vi "sub vi - Read Analog All v9.5.vi"(0 "data 0":waveform(dbl)[](array[waveform]), 5 "data 1":waveform(dbl)[](array[waveform]), 7 "data 2":waveform(dbl)[](array[waveform]), 9 "AI Error":errorcluster[](array[cluster])) -> (3 "array GRAPH":dynamicdata[](array[waveform]), 4 "LAB01":T2, 6 "LAB02":T3, 8 "LAB03":T4, 10 "LAB04":T5, 13 "deg C":dbl, 14 "USB Error":bool[](array[boolean]), 15 "LAB05":T6)   [LabVIEW 2017]
uses:
  program files/Global display 3.vi
  <vilib>/measure/mascope.llb/Amplitude and Levels 1 chan.vi
  <vilib>/measure/NI_MAPro.lvlib
  <vilib>/measure/madcrms.llb/Basic Averaged DC-RMS for N Chan.vi
panel:
  in  "normalized waveform":waveform(dbl)
  in  "Tab Control":T1(tab)
  out "LAB01-2 (PF)":dbl
  out "LAB01-1 (PF)":dbl
  out "LAB01-2 (V)":dbl
  out "LAB01-2 (A)":dbl
  out "LAB01-1 (V)":dbl
  out "LAB01-1 (A)":dbl
  out "LAB01-2 (GRAPH)":dynamicdata(graph)
  out "LAB01-1 (GRAPH)":dynamicdata(graph)
  out "LAB02-2 (PF)":dbl
  out "LAB02-1 (PF)":dbl
  out "LAB02-2 (V)":dbl
  out "LAB02-2 (A)":dbl
  out "LAB02-1 (V)":dbl
  out "LAB02-1 (A)":dbl
  out "LAB02-2 (GRAPH)":dynamicdata(graph)
  out "LAB02-1 (GRAPH)":dynamicdata(graph)
  out "LAB03-2 (PF)":dbl
  out "LAB03-1 (PF)":dbl
  out "LAB03-2 (V)":dbl
  out "LAB03-2 (A)":dbl
  out "LAB03-1 (V)":dbl
  out "LAB03-1 (A)":dbl
  out "LAB03-2 (GRAPH)":dynamicdata(graph)
  out "LAB03-1 (GRAPH)":dynamicdata(graph)
  out "LAB04-2 (PF)":dbl
  out "LAB04-1 (PF)":dbl
  out "LAB04-2 (V)":dbl
  out "LAB04-2 (A)":dbl
  out "LAB04-1 (V)":dbl
  out "LAB04-1 (A)":dbl
  out "LAB04-1 (GRAPH)":dynamicdata(graph)
  out "LAB04-2 (GRAPH)":dynamicdata(graph)
  out "LAB05-2 (PF)":dbl
  out "LAB05-1 (PF)":dbl
  out "LAB05-2 (V)":dbl
  out "LAB05-2 (A)":dbl
  out "LAB05-1 (V)":dbl
  out "LAB05-1 (A)":dbl
  out "LAB05-1 (GRAPH)":dynamicdata(graph)
  out "LAB05-2 (GRAPH)":dynamicdata(graph)
  out "A1 error":errorcluster
  out "array ERROR":errorcluster[](array[cluster])
  out "AI2-OFF":waveform(dbl)[](graph)
  out "AI2-ON":waveform(dbl)[](graph)
  out "AI1-OFF":waveform(dbl)[](graph)
  out "AI1-ON":waveform(dbl)[](graph)
  out "AI0-OFF":waveform(dbl)[](graph)
  out "AI0-ON":waveform(dbl)[](graph)
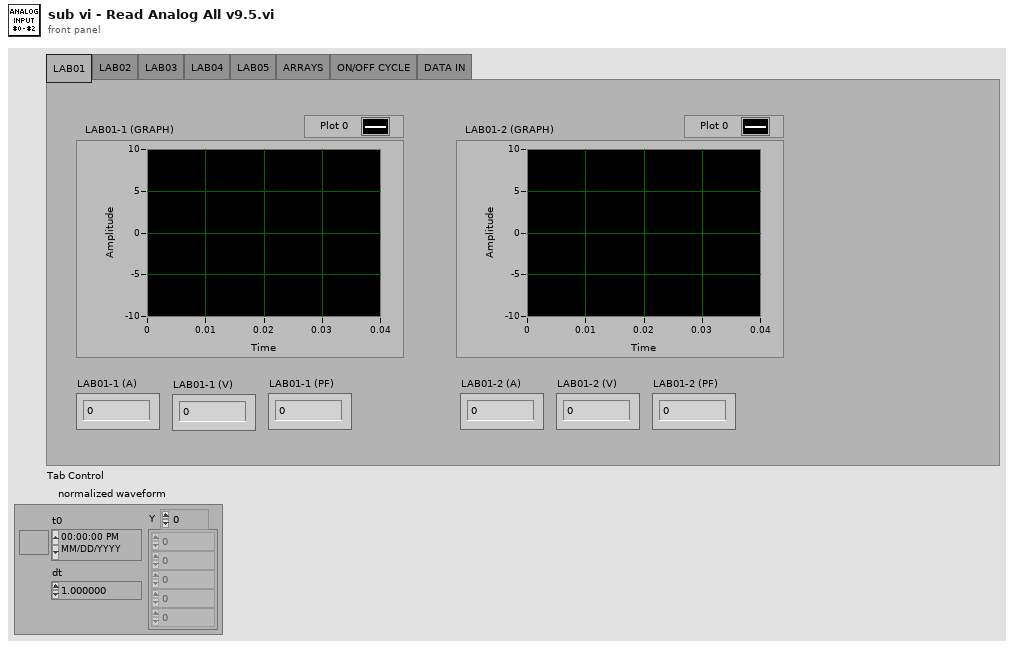
[diagram p1: front panel]
types:
  T1 = enum32{"LAB01", "LAB02", "LAB03", "LAB04", "LAB05", "ARRAYS", "ON/OFF CYCLE", "DATA IN"}
  T2 = cluster{"LAB01-1 (A)":dbl, "LAB01-1 (V)":dbl, "LAB01-1 (PF)":dbl, "LAB01-2 (A)":dbl, "LAB01-2 (V)":dbl, "LAB01-2 (PF)":dbl}
  T3 = cluster{"LAB02-1 (A)":dbl, "LAB02-1 (V)":dbl, "LAB02-1 (PF)":dbl, "LAB02-2 (A)":dbl, "LAB02-2 (V)":dbl, "LAB02-2 (PF)":dbl}
  T4 = cluster{"LAB03-1 (A)":dbl, "LAB03-1 (V)":dbl, "LAB03-1 (PF)":dbl, "LAB03-2 (A)":dbl, "LAB03-2 (V)":dbl, "LAB03-2 (PF)":dbl}
  T5 = cluster{"LAB04-1 (A)":dbl, "LAB04-1 (V)":dbl, "LAB04-1 (PF)":dbl, "LAB04-2 (A)":dbl, "LAB04-2 (V)":dbl, "LAB04-2 (PF)":dbl}
  T6 = cluster{"LAB05-1 (A)":dbl, "LAB05-1 (V)":dbl, "LAB05-1 (PF)":dbl, "LAB05-2 (A)":dbl, "LAB05-2 (V)":dbl, "LAB05-2 (PF)":dbl}
  T7 = cluster{"active power [W]":dbl, "apparent power [VA]":dbl, "reactive power [VAR]":dbl, "power factor":dbl}
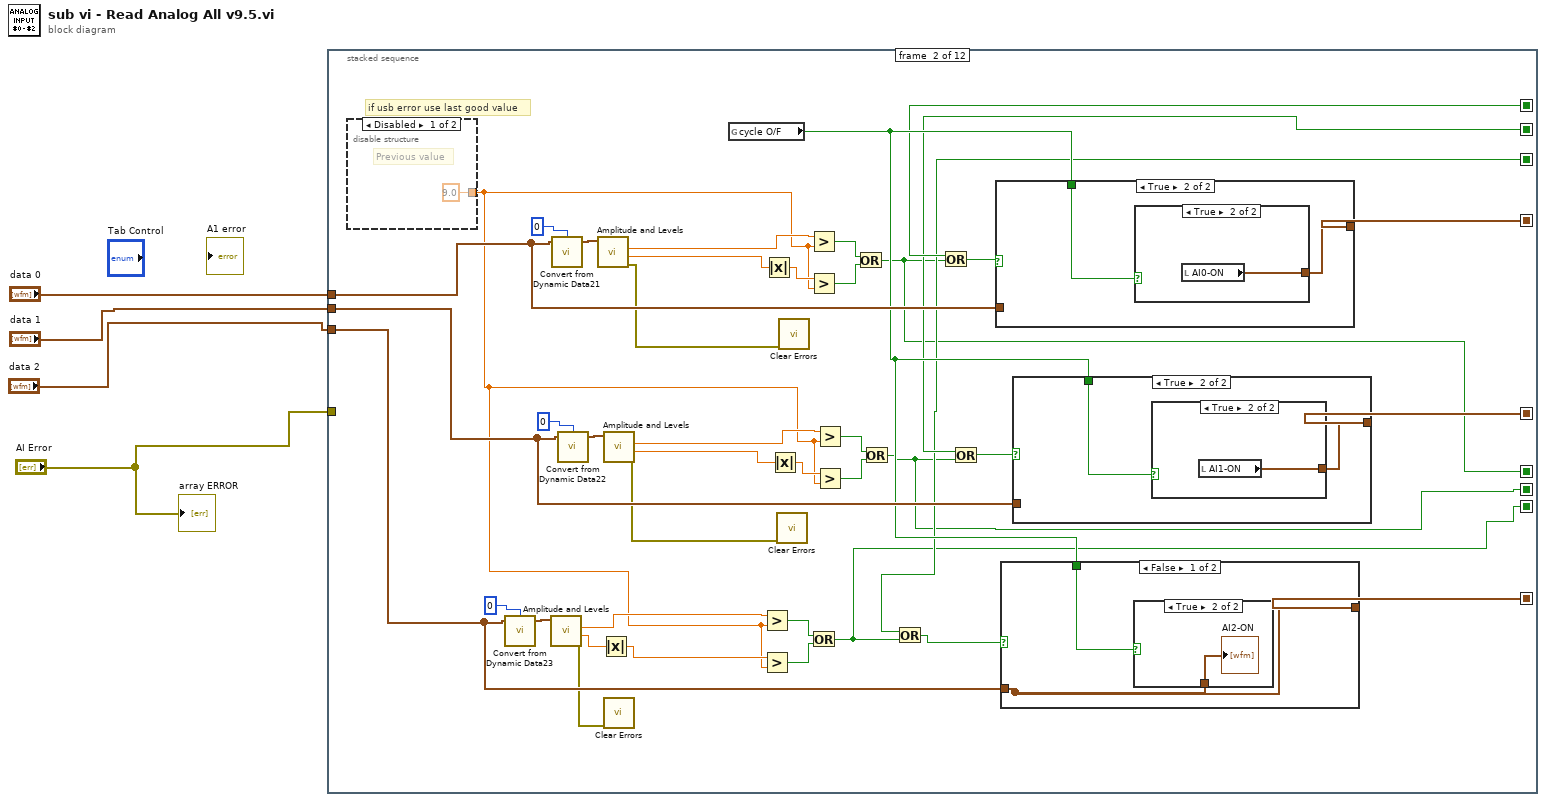
[diagram p0: block diagram]
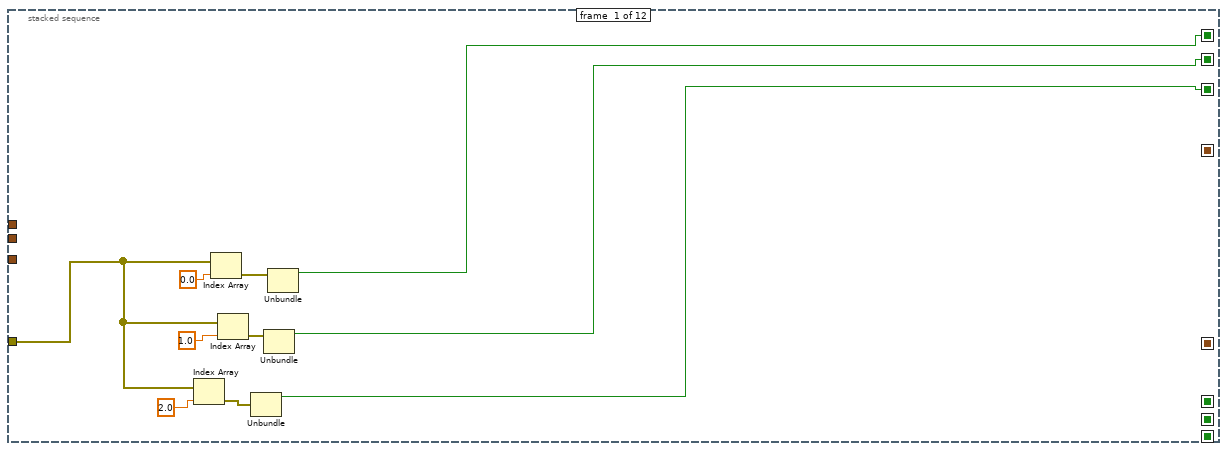
[diagram p2: hidden frame]
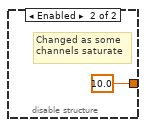
[diagram p3: hidden frame]
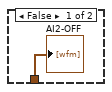
[diagram p4: hidden frame]
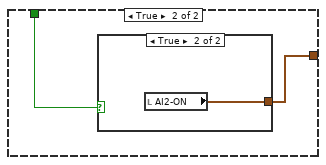
[diagram p5: hidden frame]
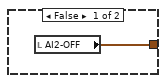
[diagram p6: hidden frame]
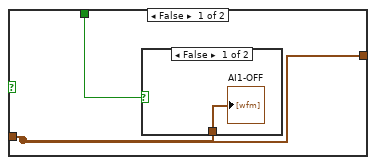
[diagram p7: hidden frame]
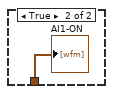
[diagram p8: hidden frame]
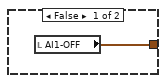
[diagram p9: hidden frame]
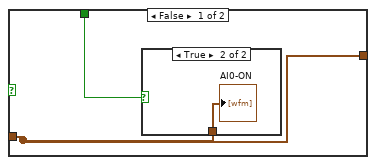
[diagram p10: hidden frame]
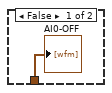
[diagram p11: hidden frame]
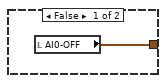
[diagram p12: hidden frame]
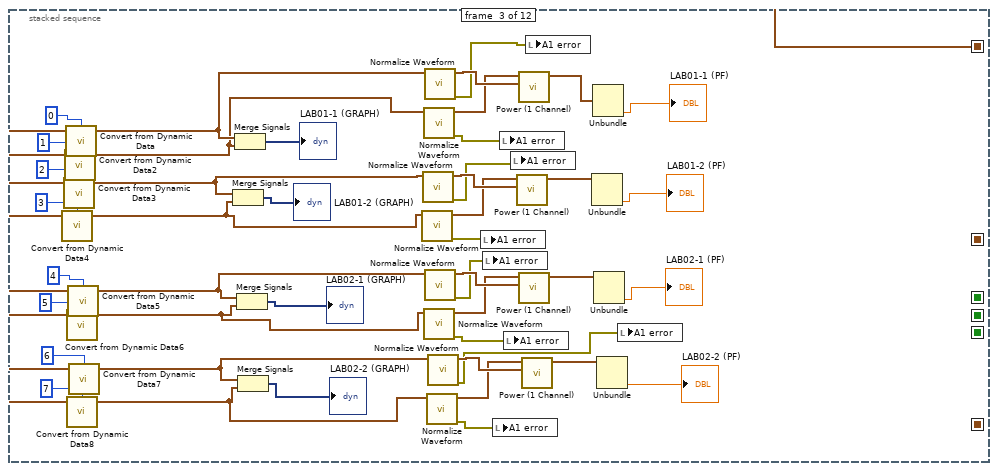
[diagram p13: hidden frame]
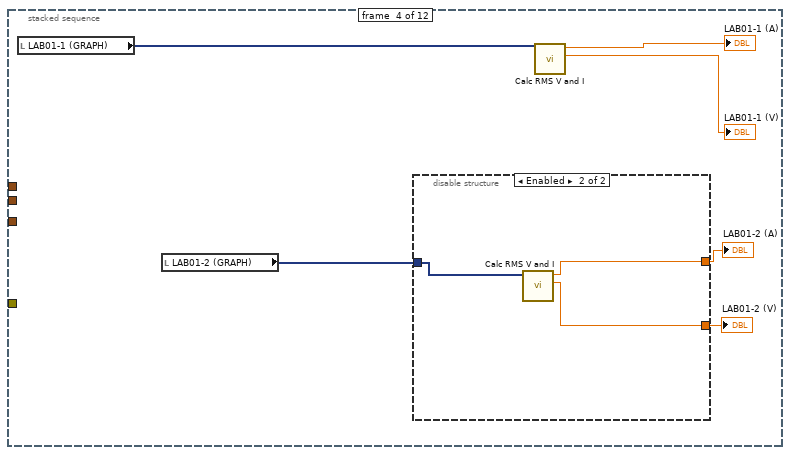
[diagram p14: hidden frame]
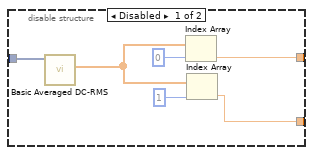
[diagram p15: hidden frame]
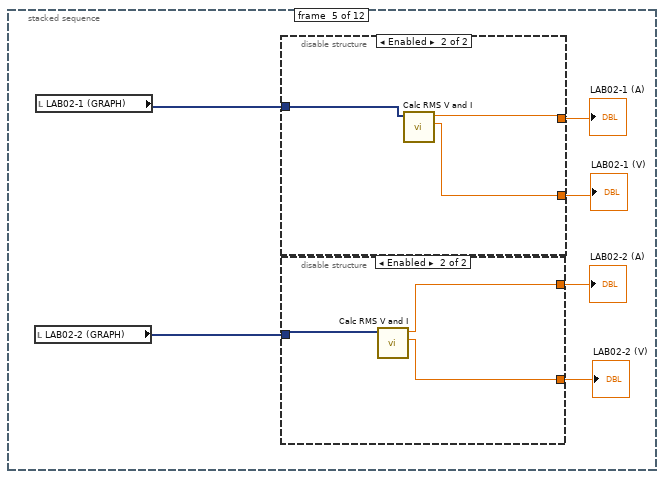
[diagram p16: hidden frame]
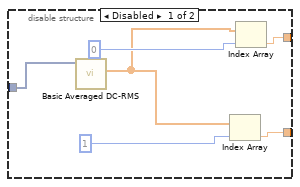
[diagram p17: hidden frame]
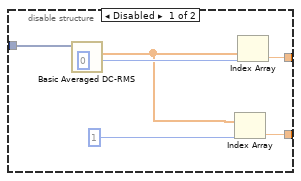
[diagram p18: hidden frame]
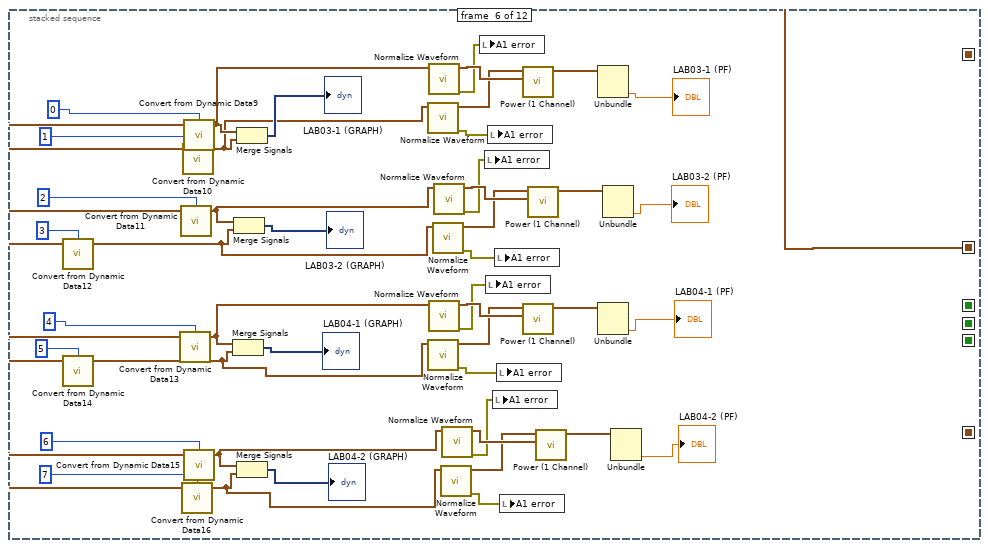
[diagram p19: hidden frame]
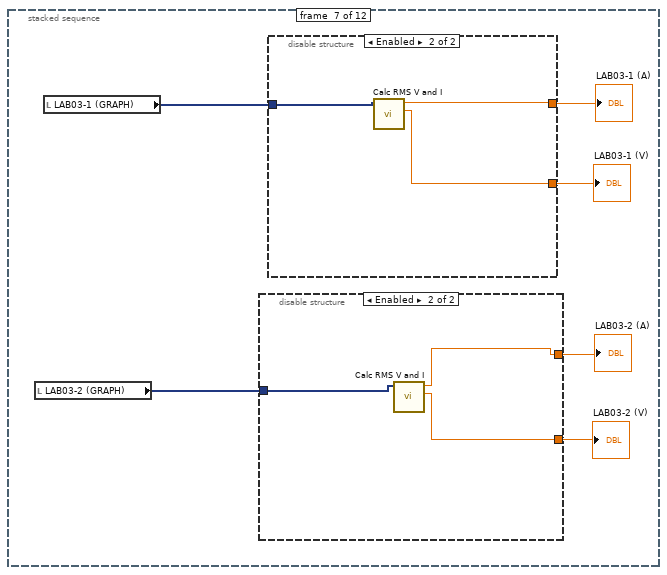
[diagram p20: hidden frame]
diagram:
  n1 = stacked-sequence {
    seq-local: [w12 _ _ _ _ _ _ _ _ _ _ _] -> [_ w22 _ _ _ _ _ _ _ _ _ w325]
    seq-local: [w9 _ _ _ _ _ _ _ _ _ _ _] -> [_ w21 _ _ _ _ _ _ _ _ _ w324]
    seq-local: [w5 _ _ _ _ _ _ _ _ _ _ _] -> [_ w18 _ _ _ _ _ _ _ _ _ w323]
    seq-local: [_ w48 _ _ _ _ _ _ _ _ _ _] -> [_ _ w126 _ _ _ _ _ _ _ _ _]
    seq-local: [_ w38 _ _ _ _ _ _ _ _ _ _] -> [_ _ _ _ _ w210 _ _ _ _ _ _]
    seq-local: [_ w27 _ _ _ _ _ _ _ _ _ _] -> [_ _ _ _ _ _ _ _ w261 _ _ _]
    seq-local: [_ w17 _ _ _ _ _ _ _ _ _ _] -> [_ _ _ _ _ _ _ _ _ _ _ w322]
    seq-local: [_ w16 _ _ _ _ _ _ _ _ _ _] -> [_ _ _ _ _ _ _ _ _ _ _ w321]
    seq-local: [_ w15 _ _ _ _ _ _ _ _ _ _] -> [_ _ _ _ _ _ _ _ _ _ _ w320]
    tunnel: "data 0" -> [_ w47 _ _ _ _ _ _ _ _ _ _]
    tunnel: "data 1" -> [_ w39 _ _ _ _ _ _ _ _ _ _]
    tunnel: "data 2" -> [_ w30 _ _ _ _ _ _ _ _ _ _]
    tunnel: "AI Error" -> [w6 _ _ _ _ _ _ _ _ _ _ _]
    frame #0 {
      n2 = Index Array(array=w6, index=2.0) -> (element=w7:errorcluster)
      n3 = Index Array(array=w6, index=0.0) -> (element=w13:errorcluster)
      n4 = Index Array(array=w6, index=1.0) -> (element=w10:errorcluster)
      n5 = Unbundle(w7) -> ("status"=w5:bool)  [unwired: 2 out]
      n6 = Unbundle(w10) -> ("status"=w9:bool)  [unwired: 2 out]
      n7 = Unbundle(w13) -> ("status"=w12:bool)  [unwired: 2 out]
    }
    frame #1 {
      # "if usb error use last good value"
      n8 = disable-structure shown="Disabled" {
        disable-tunnel: [9.0 10.0] -> w29
        frame Disabled {
          # "Previous value"
        }
        frame Enabled {
          # "Changed as some\nchannels saturate"
        }
      }
      n9 = call "Convert from Dynamic Data23"("Dynamic Data Type"=w30, "Channel"=0) -> ("Waveform"=w36:waveform(dbl))  [unwired: 2 in]
      n10 = call-poly <vilib>:"Amplitude and Levels.vi"("signal in"=w36) -> ("error out"=w24:errorcluster, "low state level"=w35:dbl, "high state level"=w34:dbl)  [unwired: 7 in, 1 out]
      n11 = call "Convert from Dynamic Data21"("Dynamic Data Type"=w47, "Channel"=0) -> ("Waveform"=w54:waveform(dbl))  [unwired: 2 in]
      n12 = call "Convert from Dynamic Data22"("Dynamic Data Type"=w39, "Channel"=0) -> ("Waveform"=w45:waveform(dbl))  [unwired: 2 in]
      n13 = call-poly <vilib>:"Amplitude and Levels.vi"("signal in"=w54) -> ("error out"=w26:errorcluster, "low state level"=w53:dbl, "high state level"=w52:dbl)  [unwired: 7 in, 1 out]
      n14 = Absolute Value(x=w35) -> (abs(x)=w33:dbl)
      n15 = call-poly <vilib>:"Amplitude and Levels.vi"("signal in"=w45) -> ("error out"=w25:errorcluster, "low state level"=w44:dbl, "high state level"=w43:dbl)  [unwired: 7 in, 1 out]
      n16 = call <vilib>:"Clear Errors.vi"("error in (no error)"=w24) -> ()  [unwired: 5 in, 2 out]
      n17 = global read "Global display 3.vi" "cycle O/F"() -> (w28:bool)
      n18 = Greater?(x=w34, y=w29) -> (0:w32:bool)
      n19 = Greater?(x=w33, y=w29) -> (0:w31:bool)
      n20 = Absolute Value(x=w53) -> (abs(x)=w51:dbl)
      n21 = Absolute Value(x=w44) -> (abs(x)=w42:dbl)
      n22 = call <vilib>:"Clear Errors.vi"("error in (no error)"=w25) -> ()  [unwired: 5 in, 2 out]
      n23 = call <vilib>:"Clear Errors.vi"("error in (no error)"=w26) -> ()  [unwired: 5 in, 2 out]
      n24 = Greater?(x=w52, y=w29) -> (0:w50:bool)
      n25 = Greater?(x=w51, y=w29) -> (0:w49:bool)
      n26 = Or(x=w32, y=w31) -> (x .or. y?=w15:bool)
      n27 = Greater?(x=w43, y=w29) -> (0:w41:bool)
      n28 = Greater?(x=w42, y=w29) -> (0:w40:bool)
      n29 = Or(x=w50, y=w49) -> (x .or. y?=w17:bool)
      n30 = Or(x=w41, y=w40) -> (x .or. y?=w16:bool)
      n31 = Or(x=w18, y=w15) -> (x .or. y?=w19:bool)
      n32 = Or(x=w22, y=w17) -> (x .or. y?=w23:bool)
      n33 = Or(x=w21, y=w16) -> (x .or. y?=w20:bool)
      n34 = case shown="True" w23 {
        tunnel: w28 -> [w75 w79]
        tunnel: [w74 w78] -> w48
        tunnel: w47 -> [w74 _]
        frame False {
          n35 = case shown="True" w75 {
            tunnel: w74 -> [w76 w77]
            frame False {
              "AI0-OFF" <- w76
            }
            frame True {
              "AI0-ON" <- w77
            }
          }
        }
        frame True {
          n36 = case shown="True" w79 {
            tunnel: [w80 w81] -> w78
            frame False {
              n37 = local read "AI0-OFF"() -> (w80:waveform(dbl)[])
            }
            frame True {
              n38 = local read "AI0-ON"() -> (w81:waveform(dbl)[])
            }
          }
        }
      }
      n39 = case shown="False" w19 {
        tunnel: w28 -> [w59 w63]
        tunnel: [w58 w62] -> w27
        tunnel: w30 -> [w58 _]
        frame False {
          n40 = case shown="True" w59 {
            tunnel: w58 -> [w60 w61]
            frame False {
              "AI2-OFF" <- w60
            }
            frame True {
              "AI2-ON" <- w61
            }
          }
        }
        frame True {
          n41 = case shown="True" w63 {
            tunnel: [w64 w65] -> w62
            frame False {
              n42 = local read "AI2-OFF"() -> (w64:waveform(dbl)[])
            }
            frame True {
              n43 = local read "AI2-ON"() -> (w65:waveform(dbl)[])
            }
          }
        }
      }
      n44 = case shown="True" w20 {
        tunnel: w28 -> [w67 w71]
        tunnel: [w66 w70] -> w38
        tunnel: w39 -> [w66 _]
        frame False {
          n45 = case shown="False" w67 {
            tunnel: w66 -> [w68 w69]
            frame False {
              "AI1-OFF" <- w68
            }
            frame True {
              "AI1-ON" <- w69
            }
          }
        }
        frame True {
          n46 = case shown="True" w71 {
            tunnel: [w72 w73] -> w70
            frame False {
              n47 = local read "AI1-OFF"() -> (w72:waveform(dbl)[])
            }
            frame True {
              n48 = local read "AI1-ON"() -> (w73:waveform(dbl)[])
            }
          }
        }
      }
    }
    frame #2 {
      n49 = call "Convert from Dynamic Data4"("Dynamic Data Type"=w126, "Channel"=3) -> ("Waveform"=w102:waveform(dbl))  [unwired: 2 in]
      n50 = call "Convert from Dynamic Data3"("Dynamic Data Type"=w126, "Channel"=2) -> ("Waveform"=w103:waveform(dbl))  [unwired: 2 in]
      n51 = call "Convert from Dynamic Data2"("Dynamic Data Type"=w126, "Channel"=1) -> ("Waveform"=w112:waveform(dbl))  [unwired: 2 in]
      n52 = call "Convert from Dynamic Data"("Dynamic Data Type"=w126, "Channel"=0) -> ("Waveform"=w113:waveform(dbl))  [unwired: 2 in]
      n53 = call "Convert from Dynamic Data6"("Dynamic Data Type"=w126, "Channel"=5) -> ("Waveform"=w97:waveform(dbl))  [unwired: 2 in]
      n54 = call "Convert from Dynamic Data8"("Dynamic Data Type"=w126, "Channel"=7) -> ("Waveform"=w91:waveform(dbl))  [unwired: 2 in]
      n55 = call "Convert from Dynamic Data5"("Dynamic Data Type"=w126, "Channel"=4) -> ("Waveform"=w98:waveform(dbl))  [unwired: 2 in]
      n56 = call "Convert from Dynamic Data7"("Dynamic Data Type"=w126, "Channel"=6) -> ("Waveform"=w92:waveform(dbl))  [unwired: 2 in]
      n57 = Merge Signals(w103, w102) -> (→"LAB01-2 (GRAPH)":dynamicdata)
      n58 = Merge Signals(w113, w112) -> (→"LAB01-1 (GRAPH)":dynamicdata)
      n59 = Merge Signals(w98, w97) -> (→"LAB02-1 (GRAPH)":dynamicdata)
      n60 = Merge Signals(w92, w91) -> (→"LAB02-2 (GRAPH)":dynamicdata)
      n61 = call <vilib>:"Normalize Waveform.vi"("waveform in"=w102) -> ("error out"=w86:errorcluster, "normalized waveform"=w106:waveform(dbl))  [unwired: 7 in, 2 out]
      n62 = call <vilib>:"Normalize Waveform.vi"("waveform in"=w103) -> ("error out"=w87:errorcluster, "normalized waveform"=w107:waveform(dbl))  [unwired: 7 in, 2 out]
      n63 = call <vilib>:"Normalize Waveform.vi"("waveform in"=w112) -> ("error out"=w88:errorcluster, "normalized waveform"=w110:waveform(dbl))  [unwired: 7 in, 2 out]
      n64 = call <vilib>:"Normalize Waveform.vi"("waveform in"=w97) -> ("error out"=w84:errorcluster, "normalized waveform"=w100:waveform(dbl))  [unwired: 7 in, 2 out]
      n65 = call <vilib>:"Normalize Waveform.vi"("waveform in"=w113) -> ("error out"=w89:errorcluster, "normalized waveform"=w111:waveform(dbl))  [unwired: 7 in, 2 out]
      n66 = call <vilib>:"Normalize Waveform.vi"("waveform in"=w98) -> ("error out"=w85:errorcluster, "normalized waveform"=w101:waveform(dbl))  [unwired: 7 in, 2 out]
      n67 = call <vilib>:"Normalize Waveform.vi"("waveform in"=w91) -> ("error out"=w82:errorcluster, "normalized waveform"=w94:waveform(dbl))  [unwired: 7 in, 2 out]
      n68 = call <vilib>:"Normalize Waveform.vi"("waveform in"=w92) -> ("error out"=w83:errorcluster, "normalized waveform"=w95:waveform(dbl))  [unwired: 7 in, 2 out]
      n69 = local write "A1 error"(w86) -> ()
      n70 = local write "A1 error"(w85) -> ()
      n71 = local write "A1 error"(w82) -> ()
      n72 = local write "A1 error"(w88) -> ()
      n73 = local write "A1 error"(w84) -> ()
      n74 = local write "A1 error"(w87) -> ()
      n75 = call "Power (1 Channel).vi"("current waveform"=w107, "voltage waveform"=w106) -> ("power value"=w105:T7)  [unwired: 9 in]
      n76 = call "Power (1 Channel).vi"("current waveform"=w111, "voltage waveform"=w110) -> ("power value"=w109:T7)  [unwired: 9 in]
      n77 = call "Power (1 Channel).vi"("current waveform"=w101, "voltage waveform"=w100) -> ("power value"=w99:T7)  [unwired: 9 in]
      n78 = call "Power (1 Channel).vi"("current waveform"=w95, "voltage waveform"=w94) -> ("power value"=w93:T7)  [unwired: 9 in]
      n79 = local write "A1 error"(w89) -> ()
      n80 = Unbundle(w105) -> ("power factor"=→"LAB01-2 (PF)":dbl)  [unwired: 3 out]
      n81 = Unbundle(w109) -> ("power factor"=→"LAB01-1 (PF)":dbl)  [unwired: 3 out]
      n82 = Unbundle(w99) -> ("power factor"=→"LAB02-1 (PF)":dbl)  [unwired: 3 out]
      n83 = Unbundle(w93) -> ("power factor"=→"LAB02-2 (PF)":dbl)  [unwired: 3 out]
      n84 = local write "A1 error"(w83) -> ()
    }
    frame #3 {
      n85 = local read "LAB01-1 (GRAPH)"() -> (w127:dynamicdata)
      n86 = local read "LAB01-2 (GRAPH)"() -> (w128:dynamicdata)
      n87 = disable-structure shown="Enabled" {
        disable-tunnel: [w135 w140] -> w132
        disable-tunnel: [w134 w139] -> w131
        disable-tunnel: w128 -> [w133 w141]
        frame Disabled {
          n88 = call-poly <vilib>:"Basic Averaged DC-RMS.vi"("signals in"=w133) -> ("RMS values"=w138:dbl[])  [unwired: 7 in, 3 out]
          n89 = Index Array(array=w138, index=0) -> (element=w135:dbl)
          n90 = Index Array(array=w138, index=1) -> (element=w134:dbl)
        }
        frame Enabled {
          n91 = call "Calc RMS V and I.vi"("LAB01-1 (GRAPH)"=w141) -> ("RMS V"=w139:dbl, "RMS I"=w140:dbl)  [unwired: 9 in]
        }
      }
      "LAB01-2 (A)" <- w132
      "LAB01-2 (V)" <- w131
      n92 = call "Calc RMS V and I.vi"("LAB01-1 (GRAPH)"=w127) -> ("RMS V"=→"LAB01-1 (V)":dbl, "RMS I"=→"LAB01-1 (A)":dbl)  [unwired: 9 in]
    }
    frame #4 {
      n93 = local read "LAB02-2 (GRAPH)"() -> (w143:dynamicdata)
      n94 = local read "LAB02-1 (GRAPH)"() -> (w142:dynamicdata)
      n95 = disable-structure shown="Enabled" {
        disable-tunnel: [w159 w164] -> w147
        disable-tunnel: [w158 w163] -> w146
        disable-tunnel: w142 -> [w157 w165]
        frame Disabled {
          n96 = call-poly <vilib>:"Basic Averaged DC-RMS.vi"("signals in"=w157) -> ("RMS values"=w160:dbl[])  [unwired: 7 in, 3 out]
          n97 = Index Array(array=w160, index=1) -> (element=w158:dbl)
          n98 = Index Array(array=w160, index=0) -> (element=w159:dbl)
        }
        frame Enabled {
          n99 = call "Calc RMS V and I.vi"("LAB01-1 (GRAPH)"=w165) -> ("RMS V"=w163:dbl, "RMS I"=w164:dbl)  [unwired: 9 in]
        }
      }
      "LAB02-1 (A)" <- w147
      "LAB02-1 (V)" <- w146
      n100 = disable-structure shown="Enabled" {
        disable-tunnel: [w150 w155] -> w145
        disable-tunnel: [w149 w154] -> w144
        disable-tunnel: w143 -> [w148 w156]
        frame Disabled {
          n101 = call-poly <vilib>:"Basic Averaged DC-RMS.vi"("signals in"=w148) -> ("RMS values"=w151:dbl[])  [unwired: 7 in, 3 out]
          n102 = Index Array(array=w151, index=1) -> (element=w149:dbl)
          n103 = Index Array(array=w151, index=0) -> (element=w150:dbl)
        }
        frame Enabled {
          n104 = call "Calc RMS V and I.vi"("LAB01-1 (GRAPH)"=w156) -> ("RMS V"=w154:dbl, "RMS I"=w155:dbl)  [unwired: 9 in]
        }
      }
      "LAB02-2 (A)" <- w145
      "LAB02-2 (V)" <- w144
    }
    frame #5 {
      n105 = call "Convert from Dynamic Data12"("Dynamic Data Type"=w210, "Channel"=3) -> ("Waveform"=w187:waveform(dbl))  [unwired: 2 in]
      n106 = call "Convert from Dynamic Data14"("Dynamic Data Type"=w210, "Channel"=5) -> ("Waveform"=w181:waveform(dbl))  [unwired: 2 in]
      n107 = call "Convert from Dynamic Data13"("Dynamic Data Type"=w210, "Channel"=4) -> ("Waveform"=w182:waveform(dbl))  [unwired: 2 in]
      n108 = call "Convert from Dynamic Data11"("Dynamic Data Type"=w210, "Channel"=2) -> ("Waveform"=w188:waveform(dbl))  [unwired: 2 in]
      n109 = call "Convert from Dynamic Data16"("Dynamic Data Type"=w210, "Channel"=7) -> ("Waveform"=w175:waveform(dbl))  [unwired: 2 in]
      n110 = call "Convert from Dynamic Data10"("Dynamic Data Type"=w210, "Channel"=1) -> ("Waveform"=w193:waveform(dbl))  [unwired: 2 in]
      n111 = call "Convert from Dynamic Data9"("Dynamic Data Type"=w210, "Channel"=0) -> ("Waveform"=w194:waveform(dbl))  [unwired: 2 in]
      n112 = call "Convert from Dynamic Data15"("Dynamic Data Type"=w210, "Channel"=6) -> ("Waveform"=w176:waveform(dbl))  [unwired: 2 in]
      n113 = Merge Signals(w182, w181) -> (→"LAB04-1 (GRAPH)":dynamicdata)
      n114 = Merge Signals(w188, w187) -> (→"LAB03-2 (GRAPH)":dynamicdata)
      n115 = Merge Signals(w194, w193) -> (→"LAB03-1 (GRAPH)":dynamicdata)
      n116 = Merge Signals(w176, w175) -> (→"LAB04-2 (GRAPH)":dynamicdata)
      n117 = call <vilib>:"Normalize Waveform.vi"("waveform in"=w193) -> ("error out"=w172:errorcluster, "normalized waveform"=w196:waveform(dbl))  [unwired: 7 in, 2 out]
      n118 = call <vilib>:"Normalize Waveform.vi"("waveform in"=w181) -> ("error out"=w168:errorcluster, "normalized waveform"=w184:waveform(dbl))  [unwired: 7 in, 2 out]
      n119 = call <vilib>:"Normalize Waveform.vi"("waveform in"=w194) -> ("error out"=w173:errorcluster, "normalized waveform"=w197:waveform(dbl))  [unwired: 7 in, 2 out]
      n120 = call <vilib>:"Normalize Waveform.vi"("waveform in"=w182) -> ("error out"=w169:errorcluster, "normalized waveform"=w185:waveform(dbl))  [unwired: 7 in, 2 out]
      n121 = call <vilib>:"Normalize Waveform.vi"("waveform in"=w187) -> ("error out"=w170:errorcluster, "normalized waveform"=w190:waveform(dbl))  [unwired: 7 in, 2 out]
      n122 = call <vilib>:"Normalize Waveform.vi"("waveform in"=w188) -> ("error out"=w171:errorcluster, "normalized waveform"=w191:waveform(dbl))  [unwired: 7 in, 2 out]
      n123 = call <vilib>:"Normalize Waveform.vi"("waveform in"=w175) -> ("error out"=w166:errorcluster, "normalized waveform"=w178:waveform(dbl))  [unwired: 7 in, 2 out]
      n124 = call <vilib>:"Normalize Waveform.vi"("waveform in"=w176) -> ("error out"=w167:errorcluster, "normalized waveform"=w179:waveform(dbl))  [unwired: 7 in, 2 out]
      n125 = local write "A1 error"(w173) -> ()
      n126 = local write "A1 error"(w171) -> ()
      n127 = local write "A1 error"(w169) -> ()
      n128 = local write "A1 error"(w172) -> ()
      n129 = local write "A1 error"(w167) -> ()
      n130 = local write "A1 error"(w170) -> ()
      n131 = local write "A1 error"(w168) -> ()
      n132 = local write "A1 error"(w166) -> ()
      n133 = call "Power (1 Channel).vi"("current waveform"=w197, "voltage waveform"=w196) -> ("power value"=w195:T7)  [unwired: 9 in]
      n134 = call "Power (1 Channel).vi"("current waveform"=w185, "voltage waveform"=w184) -> ("power value"=w183:T7)  [unwired: 9 in]
      n135 = call "Power (1 Channel).vi"("current waveform"=w191, "voltage waveform"=w190) -> ("power value"=w189:T7)  [unwired: 9 in]
      n136 = call "Power (1 Channel).vi"("current waveform"=w179, "voltage waveform"=w178) -> ("power value"=w177:T7)  [unwired: 9 in]
      n137 = Unbundle(w195) -> ("power factor"=→"LAB03-1 (PF)":dbl)  [unwired: 3 out]
      n138 = Unbundle(w183) -> ("power factor"=→"LAB04-1 (PF)":dbl)  [unwired: 3 out]
      n139 = Unbundle(w189) -> ("power factor"=→"LAB03-2 (PF)":dbl)  [unwired: 3 out]
      n140 = Unbundle(w177) -> ("power factor"=→"LAB04-2 (PF)":dbl)  [unwired: 3 out]
    }
    frame #6 {
      n141 = local read "LAB03-2 (GRAPH)"() -> (w211:dynamicdata)
      n142 = local read "LAB03-1 (GRAPH)"() -> (w212:dynamicdata)
      n143 = disable-structure shown="Enabled" {
        disable-tunnel: [w219 w223] -> w214
        disable-tunnel: [w218 w224] -> w213
        disable-tunnel: w211 -> [w217 w225]
        frame Disabled {
          n144 = call-poly <vilib>:"Basic Averaged DC-RMS.vi"("signals in"=w217) -> ("RMS values"=w220:dbl[])  [unwired: 7 in, 3 out]
          n145 = Index Array(array=w220, index=0) -> (element=w218:dbl)
          n146 = Index Array(array=w220, index=1) -> (element=w219:dbl)
        }
        frame Enabled {
          n147 = call "Calc RMS V and I.vi"("LAB01-1 (GRAPH)"=w225) -> ("RMS V"=w223:dbl, "RMS I"=w224:dbl)  [unwired: 9 in]
        }
      }
      "LAB03-2 (A)" <- w213
      "LAB03-2 (V)" <- w214
      n148 = disable-structure shown="Enabled" {
        disable-tunnel: [w228 w233] -> w216
        disable-tunnel: [w227 w232] -> w215
        disable-tunnel: w212 -> [w226 w234]
        frame Disabled {
          n149 = call-poly <vilib>:"Basic Averaged DC-RMS.vi"("signals in"=w226) -> ("RMS values"=w229:dbl[])  [unwired: 7 in, 3 out]
          n150 = Index Array(array=w229, index=0) -> (element=w228:dbl)
          n151 = Index Array(array=w229, index=1) -> (element=w227:dbl)
        }
        frame Enabled {
          n152 = call "Calc RMS V and I.vi"("LAB01-1 (GRAPH)"=w234) -> ("RMS V"=w232:dbl, "RMS I"=w233:dbl)  [unwired: 9 in]
        }
      }
      "LAB03-1 (A)" <- w216
      "LAB03-1 (V)" <- w215
    }
    frame #7 {
      n153 = local read "LAB04-2 (GRAPH)"() -> (w235:dynamicdata)
      n154 = local read "LAB04-1 (GRAPH)"() -> (w236:dynamicdata)
      n155 = disable-structure shown="Enabled" {
        disable-tunnel: [w243 w247] -> w238
        disable-tunnel: [w242 w248] -> w237
        disable-tunnel: w235 -> [w241 w249]
        frame Disabled {
          n156 = call-poly <vilib>:"Basic Averaged DC-RMS.vi"("signals in"=w241) -> ("RMS values"=w244:dbl[])  [unwired: 7 in, 3 out]
          n157 = Index Array(array=w244, index=0) -> (element=w242:dbl)
          n158 = Index Array(array=w244, index=1) -> (element=w243:dbl)
        }
        frame Enabled {
          n159 = call "Calc RMS V and I.vi"("LAB01-1 (GRAPH)"=w249) -> ("RMS V"=w247:dbl, "RMS I"=w248:dbl)  [unwired: 9 in]
        }
      }
      "LAB04-2 (A)" <- w237
      "LAB04-2 (V)" <- w238
      n160 = disable-structure shown="Enabled" {
        disable-tunnel: [w252 w257] -> w240
        disable-tunnel: [w251 w256] -> w239
        disable-tunnel: w236 -> [w250 w258]
        frame Disabled {
          n161 = call-poly <vilib>:"Basic Averaged DC-RMS.vi"("signals in"=w250) -> ("RMS values"=w253:dbl[])  [unwired: 7 in, 3 out]
          n162 = Index Array(array=w253, index=0) -> (element=w252:dbl)
          n163 = Index Array(array=w253, index=1) -> (element=w251:dbl)
        }
        frame Enabled {
          n164 = call "Calc RMS V and I.vi"("LAB01-1 (GRAPH)"=w258) -> ("RMS V"=w256:dbl, "RMS I"=w257:dbl)  [unwired: 9 in]
        }
      }
      "LAB04-1 (A)" <- w240
      "LAB04-1 (V)" <- w239
    }
    frame #8 {
      n165 = call "Convert from Dynamic Data18"("Dynamic Data Type"=w261, "Channel"=1) -> ("Waveform"=w275:waveform(dbl))  [unwired: 2 in]
      n166 = call "Convert from Dynamic Data20"("Dynamic Data Type"=w261, "Channel"=3) -> ("Waveform"=w269:waveform(dbl))  [unwired: 2 in]
      n167 = call "Convert from Dynamic Data17"("Dynamic Data Type"=w261, "Channel"=0) -> ("Waveform"=w276:waveform(dbl))  [unwired: 2 in]
      n168 = call "Convert from Dynamic Data19"("Dynamic Data Type"=w261, "Channel"=2) -> ("Waveform"=w270:waveform(dbl))  [unwired: 2 in]
      n169 = Merge Signals(w276, w275) -> (→"LAB05-1 (GRAPH)":dynamicdata)
      n170 = Merge Signals(w270, w269) -> (→"LAB05-2 (GRAPH)":dynamicdata)
      n171 = call "Convert from Dynamic Data24"("Dynamic Data Type"=w261, "Channel"=4) -> ("Waveform"=w260:waveform(dbl))  [unwired: 2 in]
      n172 = call "RMS.vi"("current waveform"=w260) -> ("RMS"=→"deg C":dbl)  [unwired: 10 in]
      n173 = call <vilib>:"Normalize Waveform.vi"("waveform in"=w275) -> ("error out"=w267:errorcluster, "normalized waveform"=w277:waveform(dbl))  [unwired: 7 in, 2 out]
      n174 = call <vilib>:"Normalize Waveform.vi"("waveform in"=w276) -> ("error out"=w266:errorcluster, "normalized waveform"=w278:waveform(dbl))  [unwired: 7 in, 2 out]
      n175 = call <vilib>:"Normalize Waveform.vi"("waveform in"=w269) -> ("error out"=w265:errorcluster, "normalized waveform"=w272:waveform(dbl))  [unwired: 7 in, 2 out]
      n176 = call <vilib>:"Normalize Waveform.vi"("waveform in"=w270) -> ("error out"=w264:errorcluster, "normalized waveform"=w273:waveform(dbl))  [unwired: 7 in, 2 out]
      n177 = local write "A1 error"(w265) -> ()
      n178 = local write "A1 error"(w266) -> ()
      n179 = local write "A1 error"(w264) -> ()
      n180 = call "Power (1 Channel).vi"("current waveform"=w278, "voltage waveform"=w277) -> ("power value"=w262:T7)  [unwired: 9 in]
      n181 = local write "A1 error"(w267) -> ()
      n182 = call "Power (1 Channel).vi"("current waveform"=w273, "voltage waveform"=w272) -> ("power value"=w271:T7)  [unwired: 9 in]
      n183 = Unbundle By Name(w262) -> ("power factor"=→"LAB05-1 (PF)":dbl)  [unwired: 3 out]
      n184 = Unbundle(w271) -> ("power factor"=→"LAB05-2 (PF)":dbl)  [unwired: 3 out]
    }
    frame #9 {
      n185 = local read "LAB05-2 (GRAPH)"() -> (w285:dynamicdata)
      n186 = local read "LAB05-1 (GRAPH)"() -> (w286:dynamicdata)
      n187 = disable-structure shown="Enabled" {
        disable-tunnel: [w293 w298] -> w290
        disable-tunnel: [w292 w297] -> w289
        disable-tunnel: w285 -> [w291 w299]
        frame Disabled {
          n188 = call-poly <vilib>:"Basic Averaged DC-RMS.vi"("signals in"=w291) -> ("RMS values"=w294:dbl[])  [unwired: 7 in, 3 out]
          n189 = Index Array(array=w294, index=1) -> (element=w292:dbl)
          n190 = Index Array(array=w294, index=0) -> (element=w293:dbl)
        }
        frame Enabled {
          n191 = call "Calc RMS V and I.vi"("LAB01-1 (GRAPH)"=w299) -> ("RMS V"=w297:dbl, "RMS I"=w298:dbl)  [unwired: 9 in]
        }
      }
      "LAB05-2 (A)" <- w290
      "LAB05-2 (V)" <- w289
      n192 = disable-structure shown="Enabled" {
        disable-tunnel: [w302 w307] -> w288
        disable-tunnel: [w301 w306] -> w287
        disable-tunnel: w286 -> [w300 w308]
        frame Disabled {
          n193 = call-poly <vilib>:"Basic Averaged DC-RMS.vi"("signals in"=w300) -> ("RMS values"=w303:dbl[])  [unwired: 7 in, 3 out]
          n194 = Index Array(array=w303, index=1) -> (element=w301:dbl)
          n195 = Index Array(array=w303, index=0) -> (element=w302:dbl)
        }
        frame Enabled {
          n196 = call "Calc RMS V and I.vi"("LAB01-1 (GRAPH)"=w308) -> ("RMS V"=w306:dbl, "RMS I"=w307:dbl)  [unwired: 9 in]
        }
      }
      "LAB05-1 (A)" <- w288
      "LAB05-1 (V)" <- w287
    }
    frame #10 {
      n197 = local read "LAB05-1 (GRAPH)"() -> (w311:dynamicdata)
      n198 = local read "LAB05-2 (GRAPH)"() -> (w310:dynamicdata)
      n199 = local read "LAB04-2 (GRAPH)"() -> (w312:dynamicdata)
      n200 = local read "LAB02-2 (GRAPH)"() -> (w316:dynamicdata)
      n201 = local read "LAB03-1 (GRAPH)"() -> (w315:dynamicdata)
      n202 = local read "LAB04-1 (GRAPH)"() -> (w313:dynamicdata)
      n203 = local read "LAB03-2 (GRAPH)"() -> (w314:dynamicdata)
      n204 = local read "LAB02-1 (GRAPH)"() -> (w317:dynamicdata)
      n205 = local read "LAB01-2 (GRAPH)"() -> (w318:dynamicdata)
      n206 = local read "LAB01-1 (GRAPH)"() -> (w319:dynamicdata)
      n207 = Build Array(w319, w318, w317, w316, w315, w314, w313, w312, w311, w310) -> (→"array GRAPH":dynamicdata[])
    }
    frame #11 {
      n208 = local read "LAB03-2 (PF)"() -> (w344:dbl)
      n209 = local read "LAB03-1 (PF)"() -> (w347:dbl)
      n210 = local read "LAB03-1 (A)"() -> (w349:dbl)
      n211 = local read "LAB03-1 (V)"() -> (w348:dbl)
      n212 = local read "LAB03-2 (A)"() -> (w346:dbl)
      n213 = local read "LAB03-2 (V)"() -> (w345:dbl)
      n214 = local read "LAB01-1 (PF)"() -> (w354:dbl)
      n215 = local read "LAB01-2 (PF)"() -> (w351:dbl)
      n216 = local read "LAB01-1 (V)"() -> (w355:dbl)
      n217 = local read "LAB01-2 (A)"() -> (w353:dbl)
      n218 = local read "LAB01-2 (V)"() -> (w352:dbl)
      n219 = local read "LAB01-1 (A)"() -> (w356:dbl)
      n220 = Bundle("LAB03-1 (A)"=w349, "LAB03-1 (V)"=w348, "LAB03-1 (PF)"=w347, "LAB03-2 (A)"=w346, "LAB03-2 (V)"=w345, "LAB03-2 (PF)"=w344) -> (→"LAB03":T4)  [unwired: 1 in]
      n221 = local read "LAB05-2 (PF)"() -> (w330:dbl)
      n222 = local read "LAB05-1 (PF)"() -> (w333:dbl)
      n223 = Bundle("LAB01-1 (A)"=w356, "LAB01-1 (V)"=w355, "LAB01-1 (PF)"=w354, "LAB01-2 (A)"=w353, "LAB01-2 (V)"=w352, "LAB01-2 (PF)"=w351) -> (→"LAB01":T2)  [unwired: 1 in]
      n224 = local read "LAB05-2 (V)"() -> (w331:dbl)
      n225 = local read "LAB05-1 (A)"() -> (w335:dbl)
      n226 = local read "LAB05-1 (V)"() -> (w334:dbl)
      n227 = local read "LAB05-2 (A)"() -> (w332:dbl)
      n228 = local read "LAB04-1 (PF)"() -> (w341:dbl)
      n229 = local read "LAB04-2 (PF)"() -> (w338:dbl)
      n230 = local read "LAB04-1 (A)"() -> (w343:dbl)
      n231 = local read "LAB04-1 (V)"() -> (w342:dbl)
      n232 = local read "LAB04-2 (A)"() -> (w340:dbl)
      n233 = local read "LAB04-2 (V)"() -> (w339:dbl)
      n234 = local read "LAB02-2 (PF)"() -> (w358:dbl)
      n235 = local read "LAB02-1 (PF)"() -> (w361:dbl)
      n236 = local read "LAB02-2 (A)"() -> (w360:dbl)
      n237 = local read "LAB02-2 (V)"() -> (w359:dbl)
      n238 = local read "LAB02-1 (V)"() -> (w362:dbl)
      n239 = local read "LAB02-1 (A)"() -> (w363:dbl)
      n240 = Bundle("LAB05-1 (A)"=w335, "LAB05-1 (V)"=w334, "LAB05-1 (PF)"=w333, "LAB05-2 (A)"=w332, "LAB05-2 (V)"=w331, "LAB05-2 (PF)"=w330) -> (→"LAB05":T6)  [unwired: 1 in]
      n241 = Bundle("LAB04-1 (A)"=w343, "LAB04-1 (V)"=w342, "LAB04-1 (PF)"=w341, "LAB04-2 (A)"=w340, "LAB04-2 (V)"=w339, "LAB04-2 (PF)"=w338) -> (→"LAB04":T5)  [unwired: 1 in]
      n242 = Bundle("LAB02-1 (A)"=w363, "LAB02-1 (V)"=w362, "LAB02-1 (PF)"=w361, "LAB02-2 (A)"=w360, "LAB02-2 (V)"=w359, "LAB02-2 (PF)"=w358) -> (→"LAB02":T3)  [unwired: 1 in]
      n243 = Or(x=w324, y=w321) -> (x .or. y?=w326:bool)
      n244 = Or(x=w325, y=w320) -> (x .or. y?=w328:bool)
      n245 = Or(x=w323, y=w322) -> (x .or. y?=w327:bool)
      n246 = Build Array(w328, w326, w327) -> (→"USB Error":bool[])
    }
  }
  "array ERROR" <- "AI Error"
